vi "Run Server.vi"(8 "error in (no error)":errorcluster, 11 "Stop OOB Server UE":refnum<user-event>) -> (0 "error out":errorcluster)   [LabVIEW 2025, in "OOB gRPC Server.lvlib"]
uses:
  OOB gRPC Server.lvlib
  <vilib>/gRPC/LabVIEW gRPC Servicer/ServiceBase/ServiceBase.lvclass
  <vilib>/gRPC/LabVIEW gRPC Servicer/Servicer/Servicer.lvclass
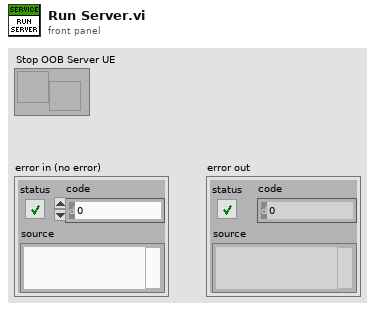
[diagram p1: front panel]
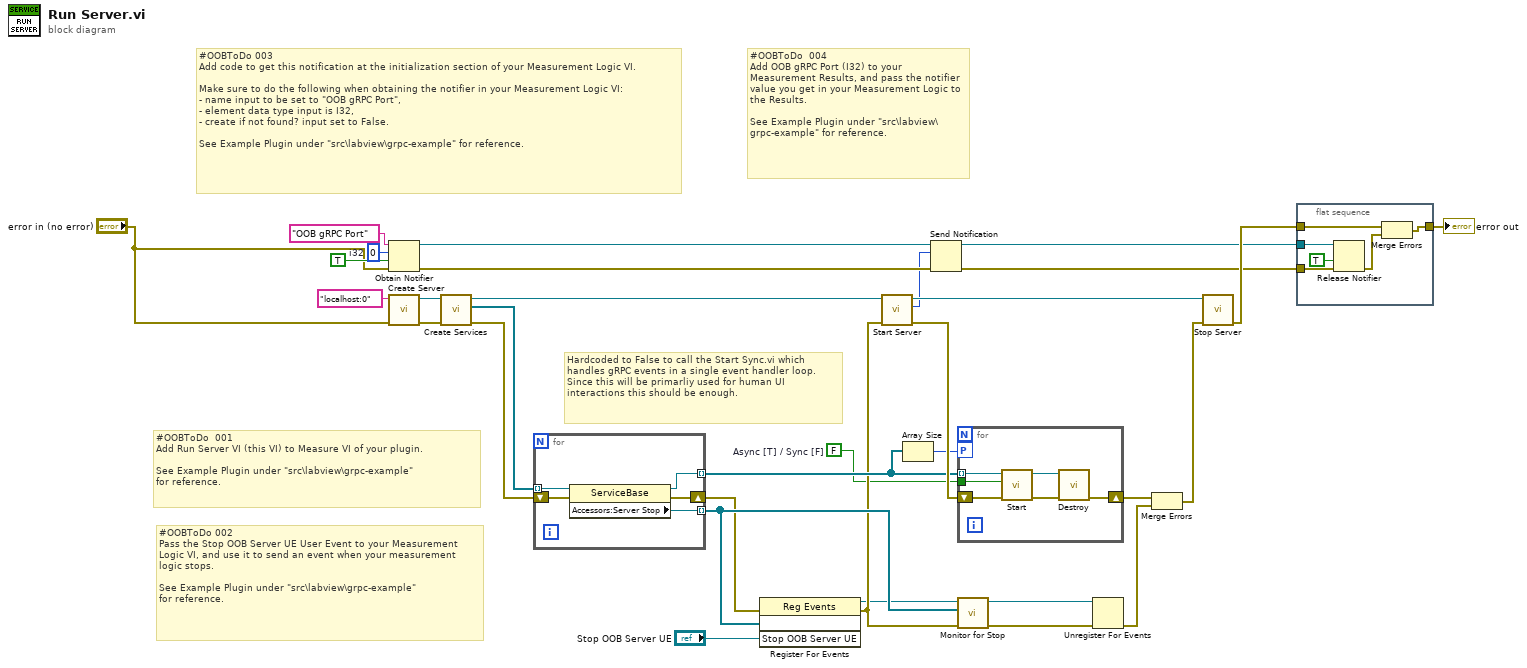
[diagram p0: block diagram]
diagram:
  w2 = FALSE  # Async [T] / Sync [F]
  w11 = 0  # i32
  # "#OOBToDo  004 \nAdd OOB gRPC Port (I32) to your Measurement Results, and pass the notifier value you get in your Measurement Logic to the Results.\n\nSee Example Plugin under \"src\\labview\\grpc-example\" for reference."
  # "#OOBToDo 002 \nPass the Stop OOB Server UE User Event to your Measurement Logic VI, and use it to send an event when your measurement logic stops.\n\nSee Example Plugin under \"src\\labview\\grpc-example\" for reference."
  # "#OOBToDo  001 \nAdd Run Server VI (this VI) to Measure VI of your plugin.\n\nSee Example Plugin under \"src\\labview\\grpc-example\" for reference."
  # "Hardcoded to False to call the Start Sync.vi which handles gRPC events in a single event handler loop.\nSince this will be primarliy used for human UI interactions this should be enough."
  # "#OOBToDo 003 \nAdd code to get this notification at the initialization section of your Measurement Logic VI. \n\nMake sure to do the following when obtaining the notifier in your Measurement Logic VI:\n- name input to be set to \"OOB gRPC Port\",\n- element data type input is I32,\n- create if not found? input set to False.\n\nSee Example Plugin under \"src\\labview\\grpc-example\" for reference."
  n1 = Obtain Notifier(name (unnamed)="OOB gRPC Port", notification data type=w11, create if not found? (T)=TRUE, error in (no error)="error in (no error)") -> (notifier out=w9:refnum<notifier>, error out=w8:errorcluster)  [unwired: 1 out]
  n2 = call <vilib>:"Create Server.vi"("error in"="error in (no error)", "Server Address"="localhost:0") -> ("error out"=w17:errorcluster, "gRPC server out"=w31:refnum<class "Servicer.lvclass">)  [unwired: 8 in]
  n3 = call "Create Services.vi"("error in (no error)"=w17, "gRPC server in"=w31) -> ("error out"=w16:errorcluster, "gRPC services out"=w15:refnum<class "ServiceBase.lvclass">[], "gRPC server out"=w30:refnum<class "Servicer.lvclass">)  [unwired: 7 in]
  n4 = for {
    tunnel: [w36] -> w26 mode=indexing
    shift-right: [w35] -> w25
    shift-left: w16 -> [w33]
    tunnel: [w37] -> w27 mode=indexing
    tunnel: w15 -> [w34] mode=indexing
    n5 = property class="ServiceBase"(reference=w34, error in=w33) -> (reference out=w37:refnum<class "ServiceBase.lvclass">, error out=w35:errorcluster, "Accessors:Server Stop"=w36:refnum<user-event>)
  }
  n6 = register-events(error in=w25, w26, "Stop OOB Server UE") -> (reference out=w1:refnum<event-registration>, error out=w24:errorcluster)  [unwired: 1 in]
  n7 = call <vilib>:"Start Server.vi"("error in"=w24, "gRPC server in"=w30) -> ("error out"=w29:errorcluster, "Listening Port"=w5:i32, "gRPC server out"=w32:refnum<class "Servicer.lvclass">)  [unwired: 7 in]
  n8 = Array Size(array=w27) -> (size(s)=w28:i32)
  n9 = Send Notification(notification=w5, notifier=w9, error in (no error)=w8) -> (notifier out=w4:refnum<notifier>, error out=w3:errorcluster)
  n10 = for {
    tunnel: w27 -> [w41] mode=indexing
    tunnel: w2 -> [w39]
    workers-P: w28 -> [_]
    shift-right: [w38] -> w23
    shift-left: w29 -> [w40]
    n11 = call-dynamic "Start.vi"("error in"=w40, "ASync [T]"=w39, "gRPC service in"=w41) -> ("error out"=w42:errorcluster, "gRPC service out"=w43:refnum<class "ServiceBase.lvclass">)  [unwired: 7 in]
    n12 = call-dynamic "Destroy.vi"("error in"=w42, "gRPC service in"=w43) -> ("error out"=w38:errorcluster)  [unwired: 8 in, 1 out]
  }
  n13 = call "Monitor for Stop.vi"("error in (no error)"=w24, "service stop events"=w26, "Event Registration Refnum in"=w1) -> ("error out"=w19:errorcluster, "Event Registration Refnum out"=w21:refnum<event-registration>)  [unwired: 7 in]
  n14 = Unregister For Events(event registration refnum=w21, error in=w19) -> (error out=w20:errorcluster)
  n15 = Merge Errors(w23, w20) -> (w22:errorcluster)
  n16 = call <vilib>:"Stop Server.vi"("error in"=w22, "gRPC server in"=w32) -> ("error out"=w18:errorcluster)  [unwired: 9 in]
  n17 = flat-sequence {
    tunnel: w4 -> [w49]
    tunnel: w18 -> [w47]
    tunnel: [w46] -> w13
    tunnel: w3 -> [w44]
    frame #0 {
      n18 = Release Notifier(notifier=w49, force destroy? (F)=TRUE, error in (no error)=w44) -> (error out=w45:errorcluster)  [unwired: 2 out]
      n19 = Merge Errors(w47, w45) -> (w46:errorcluster)
    }
  }
  "error out" <- w13
